vi "Close.vi"(8 "error in (no error)":errorcluster, 11 "WindowFrame in":refnum<class "WindowFrame.lvclass">) -> (0 "error out":errorcluster)   [LabVIEW 2021, in "WindowFrame.lvlib" / "WindowFrame.lvclass"]
uses:
  WindowFrame.lvclass
  C:/GitHub/ClassUtilities/src/ClassByRef/ClassByRef.lvclass
  ClassUtilities/src/ClassByRef/ClassByRef.lvclass/ClassByRef.ctl
  WindowFrame.lvclass/WindowFrame.ctl
  c2bc72a3-1a9b-4e60-beb5-0e1a116419cb.vi
  544d21e6-f9ca-4740-9345-a20cce9e5187.vi
  ClassUtilities/src/ClassByRef/GetRef.vi
  ClassUtilities/src/ClassByRef/CreateNotifier.vi
  ClassUtilities/src/ClassByRef/SendExitEvent.vi
  ClassUtilities/src/ClassByRef/WaitNotification.vi
  ClassUtilities/src/ClassByRef/SetNotifier.vi
  ClassUtilities/src/ClassByRef/GetExitEvent.vi
  ClassUtilities/src/ClassByRef/GetNotifier.vi
  ClassUtilities/src/ClassByRef/SetNotifier.vi/6a7be9d6-cac5-4ac9-b7fd-da113b1d2d73.vi
  ClassUtilities/src/ClassByRef/GetExitEvent.vi/d78f5ac1-b881-48f7-a86d-8a9fda2b8e49.vi
  ClassUtilities/src/ClassByRef/GetNotifier.vi/815770e3-f244-4544-877a-43bf45f14863.vi
  <vilib>/Utility/error.llb/Error Cluster From Error Code.vi
  ClassUtilities/src/ClassByRef/ClassByRef.lvclass
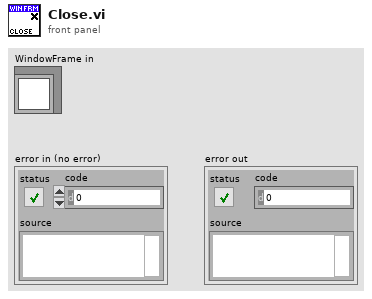
[diagram p1: front panel]
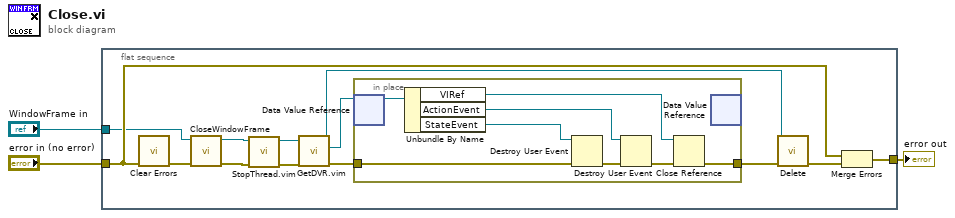
[diagram p0: block diagram]
diagram:
  n1 = flat-sequence {
    tunnel: [w15] -> w1
    tunnel: "error in (no error)" -> [w14]
    tunnel: "WindowFrame in" -> [w13]
    frame #0 {
      n2 = call <vilib>:"Clear Errors.vi"("error in (no error)"=w14) -> ("error out"=w16:errorcluster)  [unwired: 5 in, 1 out]
      n3 = call "CloseWindowFrame.vi"("error in (no error)"=w16, "WindowFrame in"=w13) -> ("error out"=w9:errorcluster, "WindowFrame out"=w8:refnum<class "WindowFrame.lvclass">)  [unwired: 8 in]
      n4 = call "StopThread.vim"("error in (no error)"=w9, "ByRefClass in"=w8) -> ("error out"=w6:errorcluster, "ByRefClass out"=w7:refnum<class "WindowFrame.lvclass">)  [unwired: 8 in]
      n5 = call "GetDVR.vim"("error in (no error)"=w6, "ByRefClass in"=w7) -> ("error out"=w5:errorcluster, "DVR"=w4:refnum<data-value>, "ByRefClass out"=w10:refnum<class "WindowFrame.lvclass">)  [unwired: 7 in]
      n6 = in-place {
        in-place-border: [w21] -> w12
        in-place-border: w5 -> [w18]
        n7 = in-place-dvr #1(w4) -> (w17:refnum<class "WindowFrame.lvclass">)  [unwired: 1 out]
        n8 = Unbundle By Name(w17) -> ("VIRef"=w20:refnum<vi>, "ActionEvent"=w22:refnum<user-event>, "StateEvent"=w24:refnum<user-event>)
        n9 = Destroy User Event(user event=w24, error in=w18) -> (error out=w23:errorcluster)
        n10 = Destroy User Event(user event=w22, error in=w23) -> (error out=w19:errorcluster)
        n11 = Close Reference(reference=w20, error in (no error)=w19) -> (error out=w21:errorcluster)
        n12 = in-place-dvr #1() -> ()  [unwired: 1 in, 2 out]
      }
      n13 = call-dynamic "Delete.vi"("error in (no error)"=w12, "ByRefClass in"=w10) -> ("error out"=w11:errorcluster)  [unwired: 8 in, 1 out]
      n14 = Merge Errors(w14, w11) -> (w15:errorcluster)
    }
  }
  "error out" <- w1
